vi "Read Command.vi"(8 "error in (no error)":errorcluster, 10 "timeout ms (5000)":i32=5000, 11 "Websocket Client Handler in":refnum<class "Websocket Client Handler.lvclass">) -> (0 "error out":errorcluster, 3 "Websocket Client Handler out":refnum<class "Websocket Client Handler.lvclass">)   [LabVIEW 2016, in "Stream Mediator.lvlib" / "Websocket Client Handler.lvclass"]
doc: "--\nCopyright © 2017 Composed SystemsI All rights reserved.\n\nAuthor: Jon McBee <jon.mcbee@composed.io>\n\nThis library is provided \"AS IS\" ,WITHOUT WARRANTIES OR\nCONDITIONS OF ANY KIND, either express or implied.\n\nComposed Systems -- composed.io\n\nStream 0.0.1.1\nJon McBee - Composed Systems\nCopyright (c) 2017, Composed Systems"
uses:
  <userlib>/Composed Systems/Stream/Mediator/Classes/Websocket Client Handler Actor/Websocket Client Handler/Websocket Client Handler.lvclass
  <userlib>/Composed Systems/Stream/Mediator/Classes/Websocket Client Handler Actor/Websocket Client Handler/Websocket Client Handler.lvclass/Websocket Client Handler.ctl
  <vilib>/MediaMongrels Ltd/WebSockets/WebSockets/WebSockets.lvlib
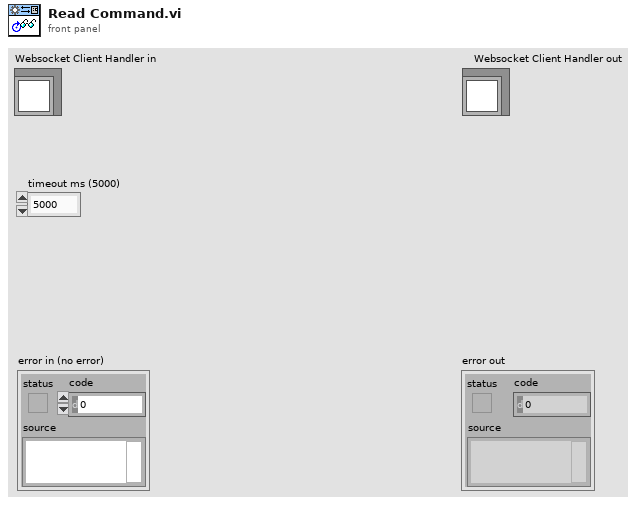
[diagram p1: front panel]
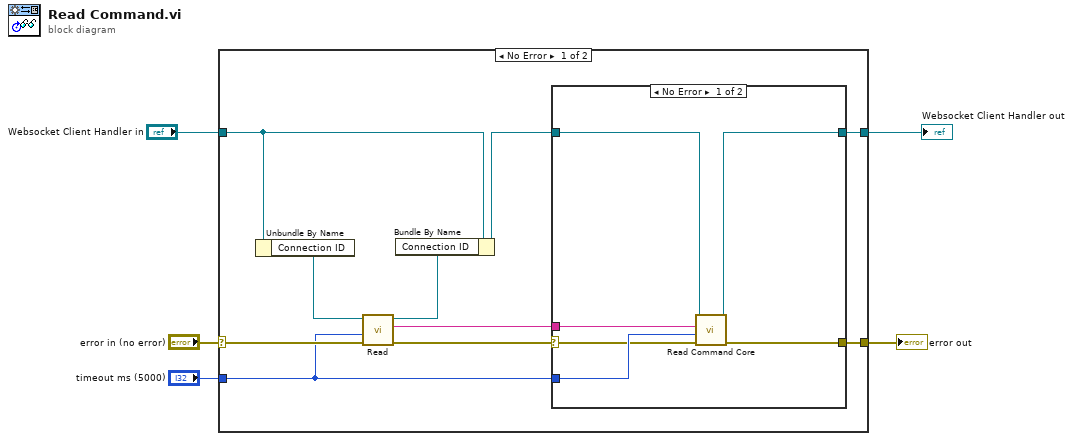
[diagram p0: block diagram]
diagram:
  n1 = case shown="No Error" "error in (no error)" {
    selector: "error in (no error)" -> [w15 w25]
    tunnel: [w12 w25] -> w4
    tunnel: "timeout ms (5000)" -> [w6 _]
    tunnel: [w11 w24] -> w2
    tunnel: "Websocket Client Handler in" -> [w8 w24]
    frame No Error {
      n2 = Unbundle By Name(w8) -> ("Connection ID"=w10:refnum<k5>)
      n3 = call <vilib>:"Read.vi"("error in (no error)"=w15, "timeout ms (5000)"=w6, "WebSocket Connection in"=w10) -> ("error out"=w13:errorcluster, "Data"=w14:string, "WebSocket Connection out"=w9:refnum<k5>)  [unwired: 5 in, 1 out]
      n4 = Bundle By Name(cluster=w8, "Connection ID"=w9) -> (w7:refnum<class "Websocket Client Handler.lvclass">)
      n5 = case shown="No Error" w13 {
        selector: w13 -> [w16 w23]
        tunnel: w14 -> [w17 _]
        tunnel: [w21 w23] -> w12
        tunnel: [w19 w22] -> w11
        tunnel: w7 -> [w20 w22]
        tunnel: w6 -> [w18 _]
        frame No Error {
          n6 = call-dynamic "Read Command Core.vi"("error in (no error)"=w16, "timeout ms (5000)"=w18, "Data"=w17, "Websocket Client Handler in"=w20) -> ("error out"=w21:errorcluster, "Websocket Client Handler out"=w19:refnum<class "Websocket Client Handler.lvclass">)  [unwired: 6 in]
        }
        frame Error {
        }
      }
    }
    frame Error {
    }
  }
  "error out" <- w4
  "Websocket Client Handler out" <- w2
